vi "S8300E_CPLD_Feature_WIH.vi"() -> ()   [LabVIEW 2011]
panel:
  out "TEMP-LOG2":string
  out "FinalLOG2":string
  out "log2":string
  out "log1":string
  out "DebugView":string
  out "CMDList":cluster{string, string, string}[](array[cluster])
  out "log msg":string
  out "VISA resource name out":refnum<visa-resource-name>
  out "BEGIN TIME":u32
  out "進行狀況":string
  # "2015-6-1"
  # "S8300E Check CPLD Feature接UART COM9)"
  # "Error Code:CPLD"
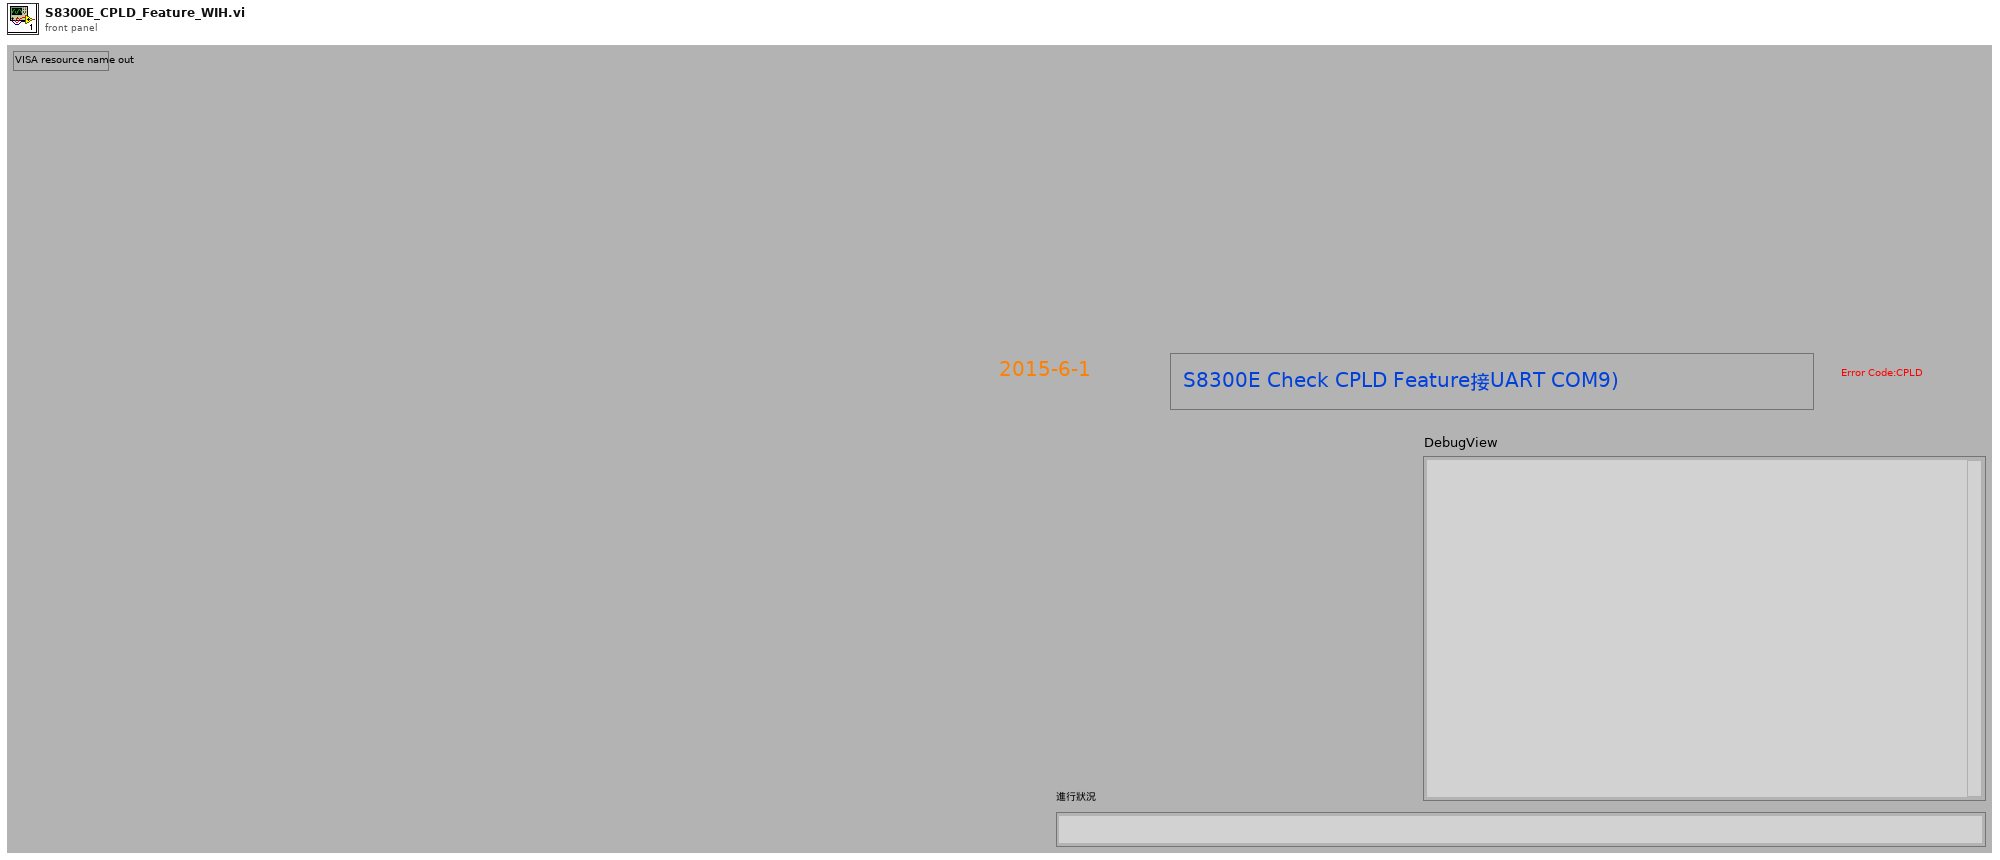
[diagram p1: front panel]
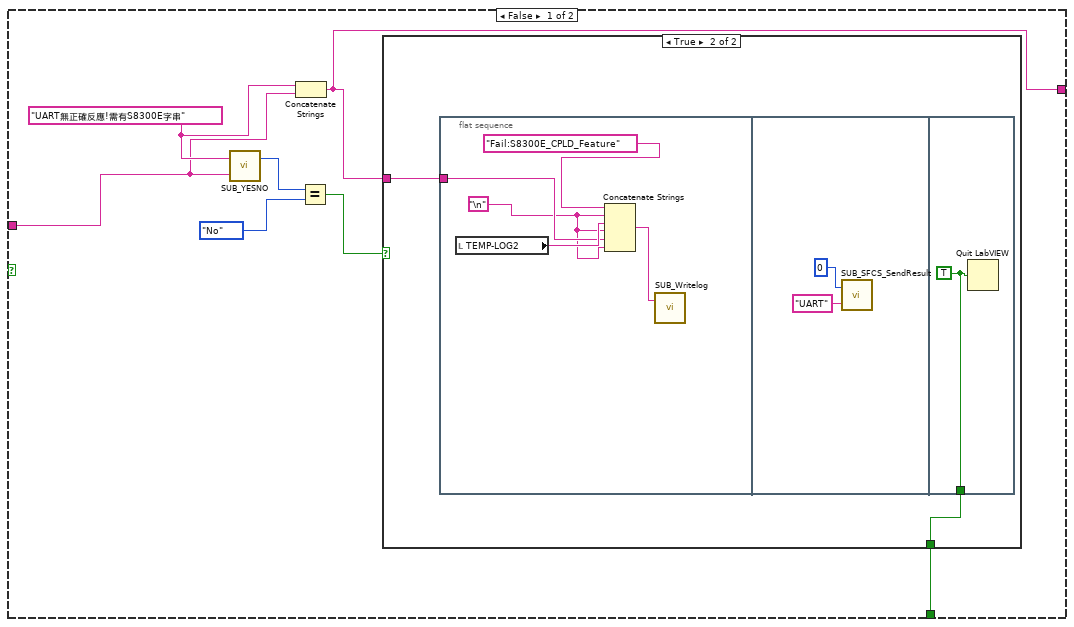
[diagram p3: hidden frame]
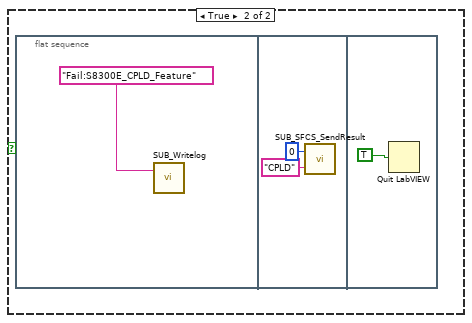
[diagram p5: hidden frame]
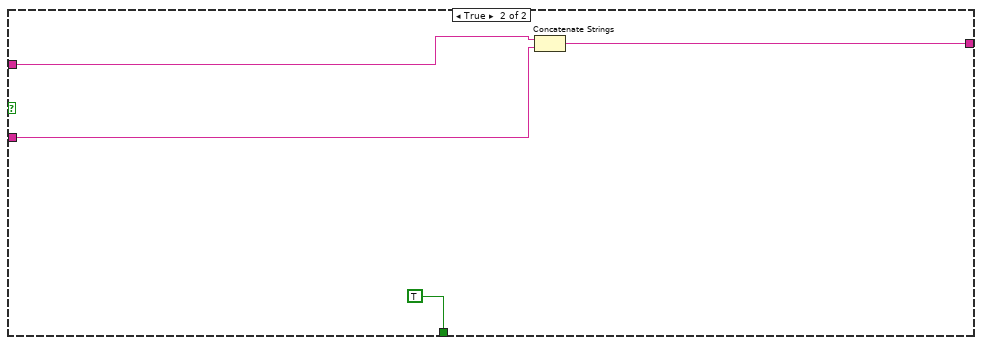
[diagram p6: hidden frame]
diagram:
  n1 = flat-sequence {
    tunnel: [w18] -> w1
    tunnel: w1 -> [w26]
    frame #0 {
      n2 = Tick Count (ms)() -> (millisecond timer value=→"BEGIN TIME":u32)
    }
    frame #1 {
      n3 = property on="進行狀況" class="Str"("Blinking"=TRUE) -> ()  [unwired: 2 in, 2 out]
      "進行狀況" <- "進入測試準備中...." ("進行狀況")
      "DebugView" <- ""
    }
    frame #2 {
      n4 = call "SUB_SearchFile_inFolder.vi"("Search Filename in Folder"="S8300E_sfcs_misc.txt") -> ("File Existing True/Flase"=w6:bool)  [unwired: 1 in]
      n5 = case shown="False" w6 {
        frame False {
          n6 = flat-sequence {
            frame #0 {
              n7 = call "Display Message to User"() -> ()  [unwired: 10 in, 2 out]
            }
            frame #1 {
              n8 = call "SUB_Writelog.vi"("Pass/Fail"="Fail:S8300E_CPLD_Feature") -> ()  [unwired: 2 in]
            }
            frame #2 {
              n9 = Quit LabVIEW(quit? (T)=TRUE) -> ()
            }
          }
        }
        frame True {
        }
      }
    }
    frame #3 {
      n10 = Concatenate Strings("./cpld.sh -t", "\r") -> (w14:string)
      n11 = Bundle(w14, "PASSED=", "CPLD Features Test") -> (w12:cluster{string, string, string})  [unwired: 1 in]
      n12 = Build Array(w12) -> (→"CMDList":cluster{string, string, string}[])
    }
    frame #4 {
      n13 = call "SUB_COM1_CLOSE.vi"("VISA resource name"=refnum<visa-resource-name> "COM9") -> ()  [unwired: 3 in]
    }
    frame #5 {
      n14 = call "SUB_COM3_INIT.vi"("baud rate (9600)"=u32 115200, "VISA resource name"=refnum<visa-resource-name> "COM9") -> ("VISA resource name out"=w18:refnum<visa-resource-name>)  [unwired: 1 out]
      "VISA resource name out" <- w18
    }
    frame #6 {
      w24 = "\r"
      n15 = Concatenate Strings(w24, w24) -> (w25:string)
      n16 = call "SUB_COM1Wrt.vi"("VISA resource name"=w26, "write buffer"=w25) -> ("duplicate VISA resource name"=w23:refnum<visa-resource-name>)  [unwired: 1 in, 1 out]
      n17 = call "SUB_ContinueCom1Read.vi"("Numeric"=1200, "duplicate VISA resource name 2"=w23) -> ("String"=w21:string)  [unwired: 1 in, 2 out]
      "log1" <- w21
      n18 = local write "DebugView"(w21) -> ()
    }
    frame #7 {
      n19 = while {
        shift-right: [w34] -> w27
        shift-left: "" -> [w33]
        stop <- w43 stop-if-true
        n20 = local read "VISA resource name out"() -> (w30:refnum<visa-resource-name>)
        n21 = Tick Count (ms)() -> (millisecond timer value=w41:u32)
        n22 = call "SUB_ContinueCom1Read.vi"("Numeric"=1200, "duplicate VISA resource name 2"=w30) -> ("duplicate VISA resource name"=w29:refnum<visa-resource-name>)  [unwired: 1 in, 2 out]
        n23 = call "SUB_COM1Wrt.vi"("VISA resource name"=w29, "write buffer"="\r") -> ("duplicate VISA resource name"=w42:refnum<visa-resource-name>)  [unwired: 1 in, 1 out]
        n24 = local read "log1"() -> (w37:string)
        n25 = call "SUB_READ_COM1_FindString_timeout.vi"("Find this String"="s8300e_func_test#", "Timeout Seccond"=3.0, "Begin time"=w41, "duplicate VISA resource name 2"=w42) -> ("Output String"=w36:string, "Found String"=w38:bool)  [unwired: 1 in, 1 out]
        n26 = Concatenate Strings(w37, w36) -> (w35:string)
        "log2" <- w35
        n27 = local write "DebugView"(w35) -> ()
        n28 = case shown="True" w38 {
          tunnel: [w48 TRUE] -> w43
          tunnel: w36 -> [w46 w62]
          tunnel: [w45 w62] -> w32
          frame False {
            w47 = "UART無正確反應!需有S8300E字串" ("Status")
            n29 = call "SUB_YESNO.vi"("Debug View"=w46, "Status"=w47) -> ("yes/no"=w51:enum32{"No Selection", "Yes", "No", "None"})  [unwired: 1 in]
            n30 = Concatenate Strings(w47, w46) -> (w45:string)
            n31 = Equal?(x=w51, y=enum32{"No Selection", "Yes", "No", "None"}."No") -> (x = y?=w49:bool)
            n32 = case shown="True" w49 {
              tunnel: [_ w53] -> w48
              tunnel: w45 -> [_ w52]
              frame False {
              }
              frame True {
                n33 = flat-sequence {
                  tunnel: w52 -> [w55]
                  tunnel: [w61] -> w53
                  frame #0 {
                    w54 = "\n"
                    n34 = local read "TEMP-LOG2"() -> (w57:string)
                    n35 = Concatenate Strings("Fail:S8300E_CPLD_Feature" ("Pass/Fail"), w54, w57, w54, w55, w54) -> (w56:string)
                    n36 = call "SUB_Writelog.vi"("Pass/Fail"=w56) -> ()  [unwired: 2 in]
                  }
                  frame #1 {
                    n37 = call "SUB_SFCS_SendResult.vi"("ErrorCode"="UART", "PASS_Fail (1/0)"=i8 0) -> ()  [unwired: 1 out]
                  }
                  frame #2 {
                    w61 = TRUE ("quit? (T)")
                    n38 = Quit LabVIEW(quit? (T)=w61) -> ()
                  }
                }
              }
            }
          }
          frame True {
          }
        }
        n39 = Concatenate Strings(w33, w32) -> (w34:string)
        "TEMP-LOG2" <- w34
      }
      "FinalLOG2" <- w27
    }
    frame #8 {
      n40 = local write "log msg"("") -> ()
    }
    frame #9 {
      n41 = local read "CMDList"() -> (w66:cluster{string, string, string}[])
      n42 = Array Size(array=w66) -> (size(s)=w68:i32)
      n43 = for {
        N: w68 -> [_]
        shift-right: [w69] -> w65
        shift-left: "" -> [w73]
        i -> [w74]
        n44 = while {
          tunnel: w74 -> [w91]
          tunnel: [w84] -> w69
          tunnel: w73 -> [w83]
          stop <- w86 stop-if-true
          n45 = local read "VISA resource name out"() -> (w76:refnum<visa-resource-name>)
          n46 = local read "CMDList"() -> (w81:cluster{string, string, string}[])
          n47 = Index Array(array=w81, index=w91) -> (element=w82:cluster{string, string, string})
          n48 = call "SUB_ContinueCom1Read.vi"("Numeric"=1200, "duplicate VISA resource name 2"=w76) -> ("duplicate VISA resource name"=w75:refnum<visa-resource-name>)  [unwired: 1 in, 2 out]
          n49 = Unbundle(w82) -> (w78:string, w79:string, w80:string)
          n50 = call "SUB_COM1Wrt.vi"("VISA resource name"=w75, "write buffer"=w78) -> ("duplicate VISA resource name"=w90:refnum<visa-resource-name>)  [unwired: 1 in, 1 out]
          n51 = Tick Count (ms)() -> (millisecond timer value=w89:u32)
          n52 = call "SUB_READ_COM1_FindString_timeout.vi"("Find this String"=w79, "Timeout Seccond"=3.0, "Begin time"=w89, "duplicate VISA resource name 2"=w90) -> ("Output String"=w85:string, "Found String"=w87:bool)  [unwired: 1 in, 1 out]
          n53 = local write "進行狀況"(w80) -> ()
          n54 = case shown="False" w87 {
            tunnel: [_ TRUE] -> w86
            tunnel: w85 -> [w97 w104]
            tunnel: [w93 w103] -> w84
            tunnel: w83 -> [w93 w102]
            frame False {
              n55 = call "SUB_YESNO.vi"("Debug View"=w97, "Status"="測試失敗!需回PASSED=" ("string")) -> ("yes/no"=w96:enum32{"No Selection", "Yes", "No", "None"})  [unwired: 1 in]
              n56 = Equal?(x=w96, y=enum32{"No Selection", "Yes", "No", "None"}."No") -> (x = y?=w94:bool)
              n57 = case shown="False" w94 {
                frame False {
                }
                frame True {
                  n58 = flat-sequence {
                    frame #0 {
                      n59 = call "SUB_Writelog.vi"("Pass/Fail"="Fail:S8300E_CPLD_Feature") -> ()  [unwired: 2 in]
                    }
                    frame #1 {
                      n60 = call "SUB_SFCS_SendResult.vi"("ErrorCode"="CPLD", "PASS_Fail (1/0)"=i8 0) -> ()  [unwired: 1 out]
                    }
                    frame #2 {
                      n61 = Quit LabVIEW(quit? (T)=TRUE) -> ()
                    }
                  }
                }
              }
            }
            frame True {
              n62 = Concatenate Strings(w102, w104) -> (w103:string)
            }
          }
        }
        n63 = local read "log2"() -> (w70:string)
        n64 = local read "log1"() -> (w72:string)
        n65 = Concatenate Strings(w72, w70, w69) -> (w71:string)
        n66 = local write "DebugView"(w71) -> ()
      }
      "log msg" <- w65
    }
    frame #10 {
      n67 = call "SUB_COM1_CLOSE.vi"("VISA resource name"=refnum<visa-resource-name> "COM9") -> ()  [unwired: 3 in]
    }
    frame #11 {
      w109 = "***Not Good ***" ("replace string (\"\")")
      w114 = "\n"
      n68 = local read "FinalLOG2"() -> (w116:string)
      n69 = local read "log msg"() -> (w115:string)
      n70 = local read "BEGIN TIME"() -> (w119:u32)
      n71 = Tick Count (ms)() -> (millisecond timer value=w118:u32)
      n72 = call "SUB_CAL_TESTTIME.vi"("Test Item name"="S8300E_CPLD_Feature", "Stop tick time"=w118, "Start tick time"=w119) -> ("Test Time output"=w113:string)  [unwired: 2 in]
      n73 = Concatenate Strings("Pass:S8300E_CPLD_Feature", w114, w116, w114, w115, w114, w113) -> (w108:string)
      n74 = call "SUB_SEARCH_REPLACE_STR.vi"("replace string (\"\")"=w109, "search string"="FAILED", "input string"=w108) -> ("result string"=w111:string)  [unwired: 2 in]
      n75 = call "SUB_SEARCH_REPLACE_STR.vi"("replace string (\"\")"=w109, "search string"="FAIL", "input string"=w111) -> ("result string"=w107:string)  [unwired: 2 in]
      n76 = call "SUB_Writelog.vi"("Pass/Fail"=w107) -> ()  [unwired: 2 in]
    }
    frame #12 {
      n77 = Request Deallocation(TRUE ("flag")) -> ()
    }
    frame #13 {
      n78 = Quit LabVIEW(quit? (T)=TRUE ("stop? (T)")) -> ()
    }
  }
